vi "PV ActiveLine - Sensor On-Off (TPG362).vi"(7 "W/R":bool, 8 "Fehler (Eingang)":errorcluster, 9 "Sensor 2 Set":u8(ring) items=["No status change", "Turn gauge off", "Turn gauge on"], 10 "Sensor 1 Set":u8(ring) items=["No status change", "Turn gauge off", "Turn gauge on"], 11 "Referenz in":refnum<visa-resource-name>) -> (0 "Cluster (Ausgang)":errorcluster, 1 "Sensor 2 Set":u8(ring) items=["Gauge cannot be turned on/off", "Gauge turned off", "Gauge turned on"], 2 "Sensor 1 Set":u8(ring) items=["Gauge cannot be turned on/off", "Gauge turned off", "Gauge turned on"], 3 "Referenz out":refnum<visa-resource-name>)   [LabVIEW 2013, in "PV ActiveLine.lvlib"]
doc: "SEN - Turning a Gauge on/off\n\nTransmit: SEN [,a,b]\n\nGauge 1,\na =\n0 –> No status change\n1 –> Turn gauge off\n2 –> Turn gauge on\n\nGauge 2,\nb=\n0 –> No status change\n1 –> Turn gauge off\n2 –> Turn gauge on"
uses:
  <instrlib>/PV ActiveLine/PV ActiveLine.lvlib
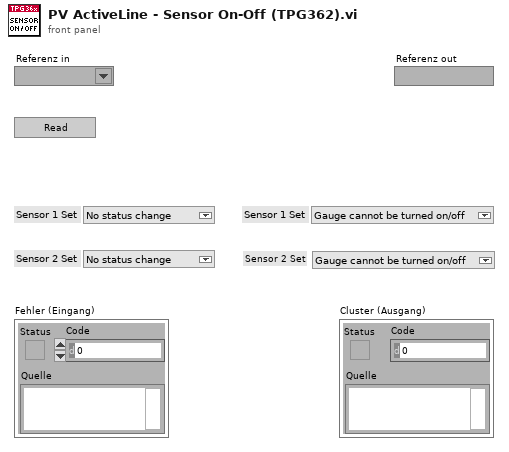
[diagram p1: front panel]
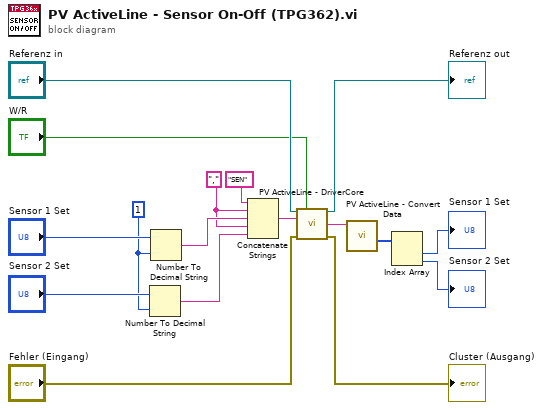
[diagram p0: block diagram]
diagram:
  w1 = i16 1 ("Breite (-)")
  w5 = ","
  n1 = Number To Decimal String(number="Sensor 2 Set", width (-)=w1) -> (decimal integer string=w4:string)
  n2 = Number To Decimal String(number="Sensor 1 Set", width (-)=w1) -> (decimal integer string=w6:string)
  n3 = Concatenate Strings("SEN", w5, w6, w5, w4) -> (w12:string)
  n4 = call <instrlib>:"PV ActiveLine - DriverCore.vi"("Referenz in"="Referenz in", "Write/Read"="W/R", "Command"=w12, "Fehler (Eingang)"="Fehler (Eingang)") -> ("Referenz out"=→"Referenz out":refnum<visa-resource-name>, "String Out"=w10:string, "Cluster (Ausgang)"=→"Cluster (Ausgang)":errorcluster)  [unwired: 9 in]
  n5 = call <instrlib>:"PV ActiveLine - Convert Data.vi"("String in"=w10) -> ("Integer Out"=w9:i32[])  [unwired: 7 in, 3 out]
  n6 = Index Array(array=w9) -> (element #1=→"Sensor 1 Set":i32, element #2=→"Sensor 2 Set":i32)  [unwired: 2 in]
